vi "write raw default value.vi"(8 "error in":errorcluster, 10 "raw default":string, 11 "system tag in":refnum<class "tag descriptor.lvclass">) -> (0 "error out":errorcluster, 3 "system tag out":refnum<class "tag descriptor.lvclass">)   [LabVIEW 2013, in "tag bus.lvlib" / "tag descriptor.lvclass"]
doc: "Writes the default value field stored in the tag descriptor. This is a raw string, not an interpreted data type."
uses:
  tag descriptor.lvclass
  tag descriptor.lvclass/tag descriptor.ctl
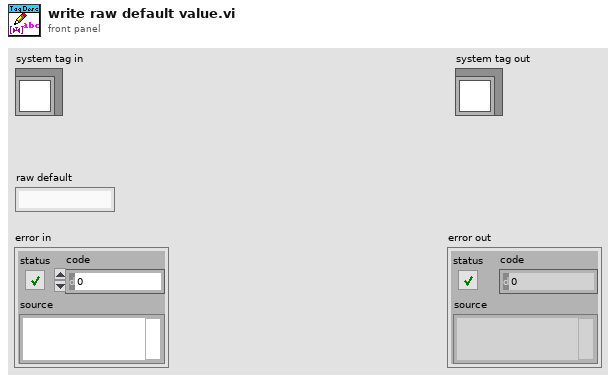
[diagram p1: front panel]
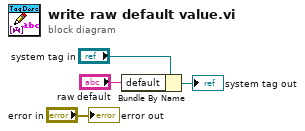
[diagram p0: block diagram]
diagram:
  n1 = Bundle By Name(cluster="system tag in", "default"="raw default") -> (→"system tag out":refnum<class "tag descriptor.lvclass">)
  "error out" <- "error in"
